vi "Dlg-Search-Stock.vi"(8 "error in (no error)":errorcluster) -> (0 "error out":errorcluster, 1 "Stock Selected":refnum<class "Stock.lvclass">, 2 "Canceled":bool, 3 "OK ?":bool)   [LabVIEW 2012]
uses:
  Stock Search.ctl
  Stock/Stock.lvclass
  Stock Manager Action.ctl
  Stock/Stock.lvclass/Stock.ctl
panel:
  in  "Stock":i32[](listbox)
  in  "Rechercher":string
  in  "Stock Search":T1
  in  "OK":bool
  out "Label":string
  in  "Cancel Button":bool
  # "Nouveau Portefeuille"
  # "Rechercher un Titre"
  # "Titre"
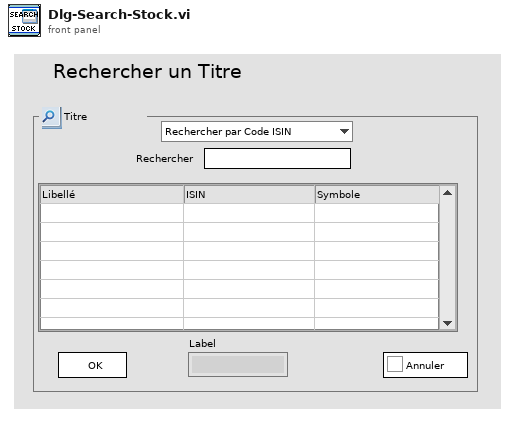
[diagram p1: front panel]
types:
  T1 = typedef "Stock Search.ctl" = enum16{"Rechercher par Code ISIN", "Rechercher par Libellé", "Rechercher par Symbole"}
  T2 = typedef "Stock Manager Action.ctl" = enum16{"Get_Stocks", "Load_Stocks", "Find_Stock_From_ISIN", "Find_Stock_From_Label", "Find_Stock_From_Symbol"}
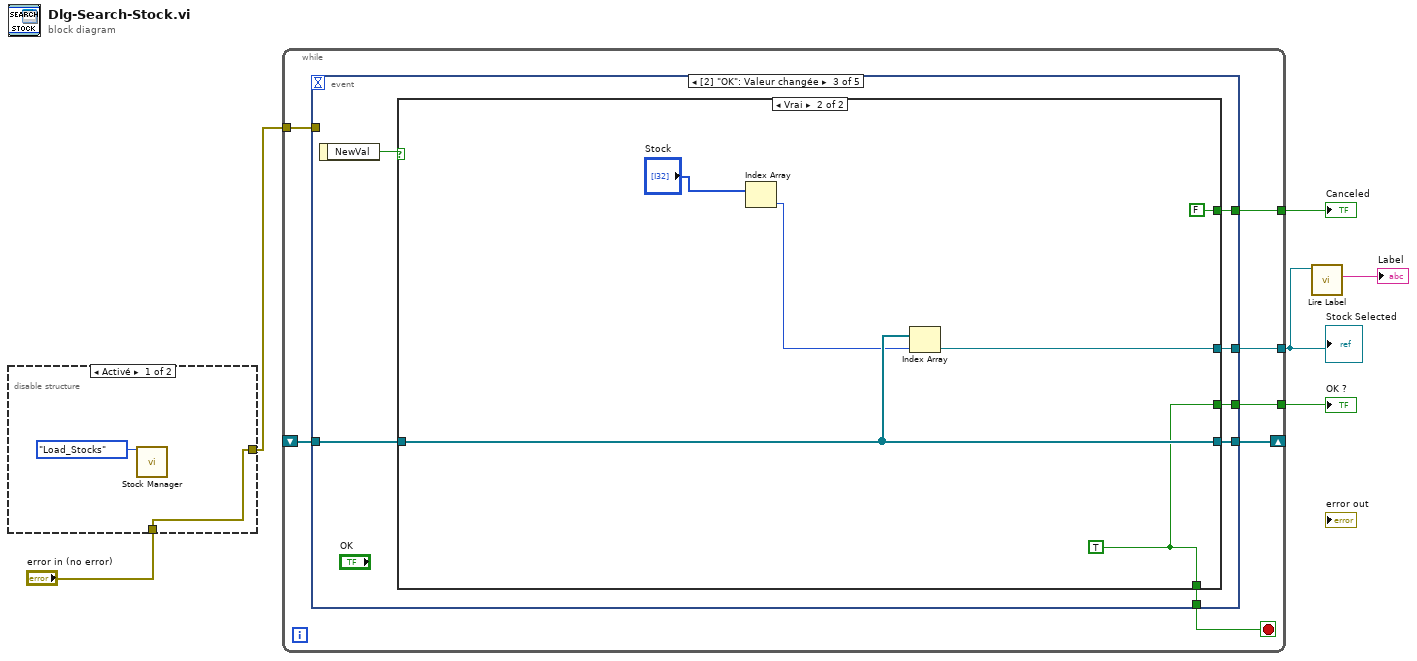
[diagram p0: block diagram]
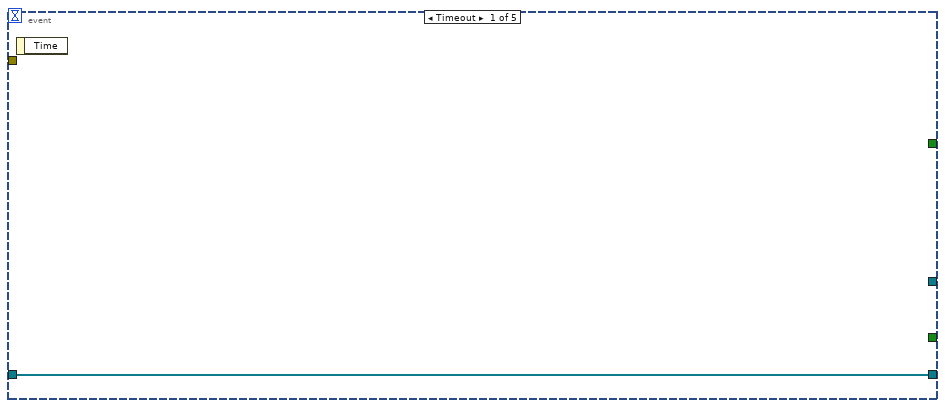
[diagram p2: hidden frame]
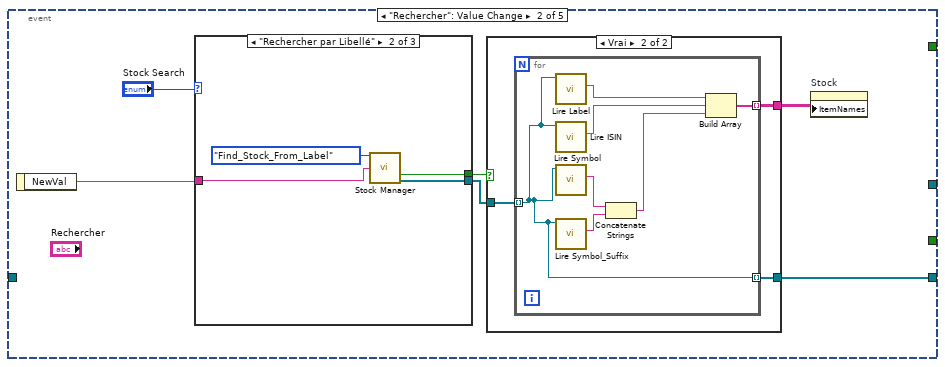
[diagram p3: hidden frame]
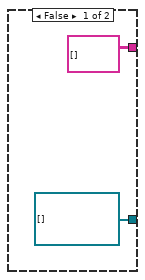
[diagram p4: hidden frame]
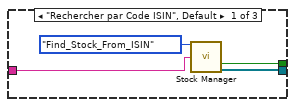
[diagram p5: hidden frame]
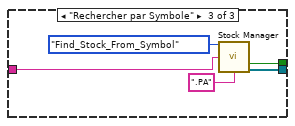
[diagram p6: hidden frame]
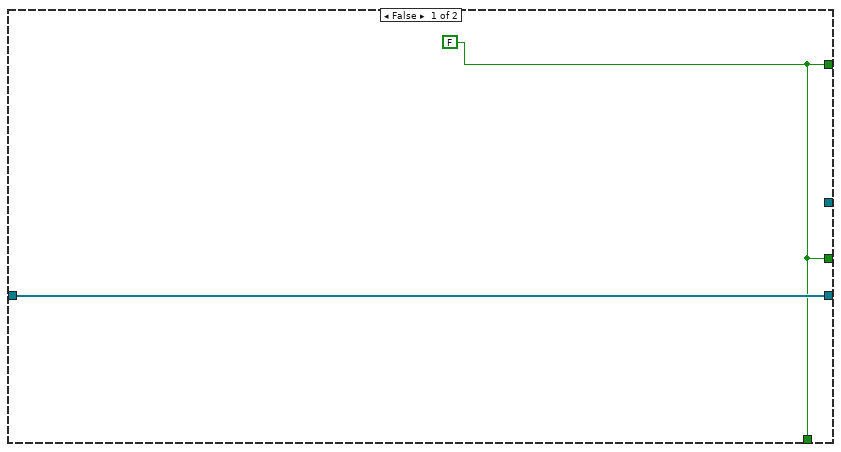
[diagram p7: hidden frame]
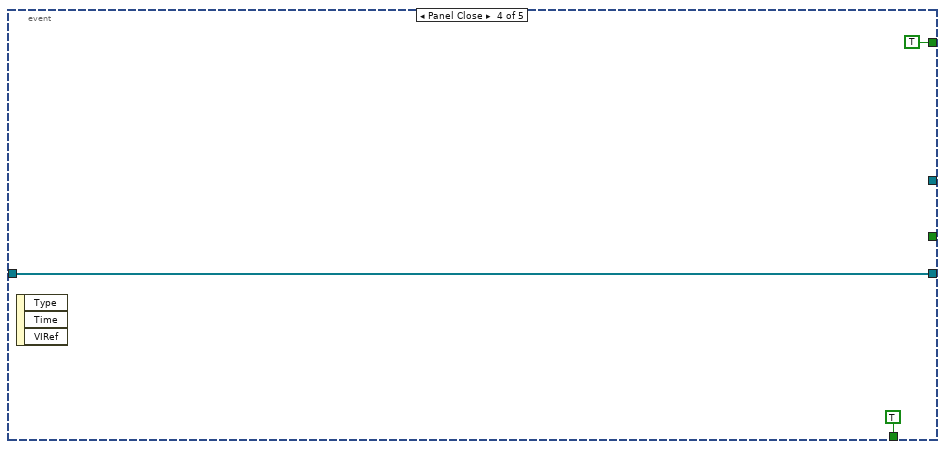
[diagram p8: hidden frame]
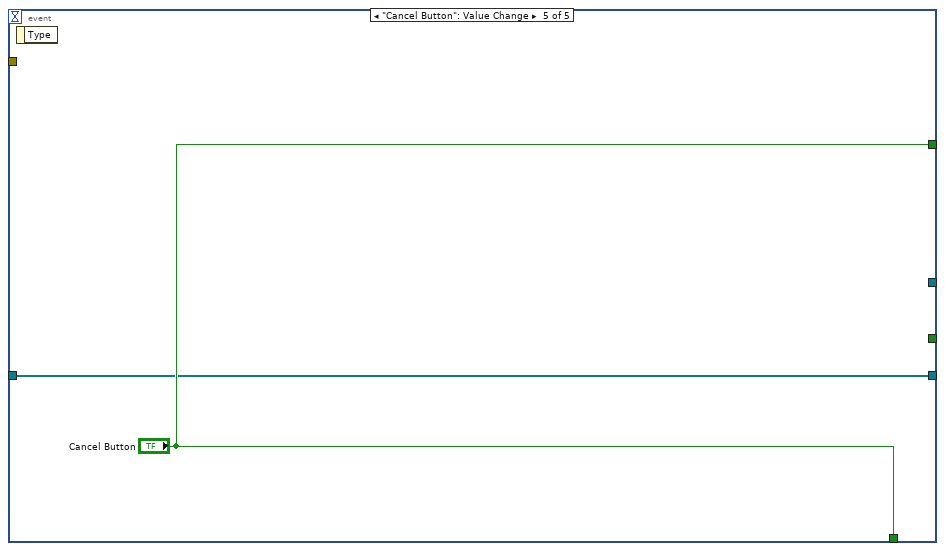
[diagram p9: hidden frame]
diagram:
  n1 = disable-structure shown="Activé" {
    disable-tunnel: [w7 _] -> w6
    disable-tunnel: "error in (no error)" -> [w7 _]
    frame Enabled {
      n2 = call "Stock Manager.vi"("Stock Manager Action"=Stock_Manager_Action."Load_Stocks") -> ()  [unwired: 12 in, 3 out]
    }
    frame Disabled {
    }
  }
  n3 = while {
    tunnel: w6 -> [w15]
    tunnel: [w14] -> w4
    shift-right: [w12] -> _
    shift-left: _ -> [w11]
    tunnel: [w10] -> w2
    tunnel: [w9] -> w3
    stop <- w13 stop-if-true
    n4 = event shown="[2] \"OK\": Valeur changée" {
      selector: _ -> [_ _ _ _ _]
      dyn-events: _ -> [_ _ _ _ _]
      timeout: _ -> [_ _ _ _ _]
      tunnel: w15 -> [_ _ _ _ _]
      tunnel: [_ _ w53 TRUE ("Cancel Button") "Cancel Button"] -> w14
      tunnel: [_ _ w52 TRUE ("Cancel Button") "Cancel Button"] -> w13
      tunnel: [w16 w17 w50 w63 w66] -> w12
      tunnel: w11 -> [w16 _ w51 w63 w66]
      tunnel: [_ _ w49 _ _] -> w10
      tunnel: [_ _ w48 _ _] -> w9
      event Timeout {
        n5 = event-data() -> ()  [unwired: 1 in, 1 out]
      }
      event "Rechercher": Value Change {
        n6 = event-data() -> ("NewVal"=w21:string)  [unwired: 1 in]
        n7 = case shown="\"Rechercher par Libellé\"" "Stock Search" {
          tunnel: w21 -> [w37 w41 w46]
          tunnel: [w36 w40 w44] -> w20
          tunnel: [w35 w39 w43] -> w19
          frame "Rechercher par Code ISIN", Default {
            n8 = call "Stock Manager.vi"("Stock Manager Action"=Stock_Manager_Action."Find_Stock_From_ISIN", "String to find (ISIN,Label,Symbol)"=w37) -> ("Stocks Found ?"=w36:bool, "Stocks Found"=w35:refnum<class "Stock.lvclass">[])  [unwired: 11 in, 1 out]
          }
          frame "Rechercher par Libellé" {
            n9 = call "Stock Manager.vi"("Stock Manager Action"=Stock_Manager_Action."Find_Stock_From_Label", "String to find (ISIN,Label,Symbol)"=w41) -> ("Stocks Found ?"=w40:bool, "Stocks Found"=w39:refnum<class "Stock.lvclass">[])  [unwired: 11 in, 1 out]
          }
          frame "Rechercher par Symbole" {
            n10 = call "Stock Manager.vi"("Stock Manager Action"=Stock_Manager_Action."Find_Stock_From_Symbol", "String to find (ISIN,Label,Symbol)"=w46, "Symbol_Suffix (.PA)"=".PA") -> ("Stocks Found ?"=w44:bool, "Stocks Found"=w43:refnum<class "Stock.lvclass">[])  [unwired: 10 in, 1 out]
          }
        }
        n11 = case shown="Vrai" w20 {
          tunnel: w19 -> [_ w27]
          tunnel: [string[][] [] w26] -> w18
          tunnel: [refnum<class "Stock.lvclass">[] [] w25] -> w17
          frame False {
          }
          frame True {
            n12 = for {
              tunnel: w27 -> [w28] mode=indexing
              tunnel: [w29] -> w26 mode=indexing
              tunnel: [w28] -> w25 mode=indexing
              n13 = call "Lire Label.vi"("Share en entrée"=w28) -> ("Label"=w32:string)  [unwired: 8 in, 2 out]
              n14 = call "Lire ISIN.vi"("Share en entrée"=w28) -> ("ISIN"=w31:string)  [unwired: 8 in, 2 out]
              n15 = call "Lire Symbol.vi"("Share en entrée"=w28) -> ("Symbol"=w34:string)  [unwired: 8 in, 2 out]
              n16 = call "Lire Symbol_Suffix.vi"("Stock en entrée"=w28) -> ("Symbol_Suffix"=w33:string)  [unwired: 8 in, 2 out]
              n17 = Concatenate Strings(w34, w33) -> (w30:string)
              n18 = Build Array(w32, w31, w30) -> (w29:string[])
            }
          }
        }
        n19 = property on="Stock" class="ListeMCol (strict)"("ItemNames"=w18) -> ()  [unwired: 2 in, 2 out]
      }
      event "OK": Value Change {
        n20 = event-data() -> ("NewVal"=w54:bool)  [unwired: 1 in]
        n21 = case shown="Vrai" w54 {
          tunnel: [w55 FALSE] -> w53
          tunnel: [w55 w57] -> w52
          tunnel: w51 -> [w56 w60]
          tunnel: [w56 w60] -> w50
          tunnel: [_ w58] -> w49
          tunnel: [w55 w57] -> w48
          frame False {
            w55 = FALSE
          }
          frame True {
            w57 = TRUE
            n22 = Index Array(array="Stock") -> (element=w59:i32)  [unwired: 1 in]
            n23 = Index Array(array=w60, index=w59) -> (element=w58:refnum<class "Stock.lvclass">)
          }
        }
      }
      event Panel Close {
        n24 = event-data() -> ()  [unwired: 1 in, 3 out]
      }
      event "Cancel Button": Value Change {
        n25 = event-data() -> ()  [unwired: 1 in, 1 out]
      }
    }
  }
  "Canceled" <- w4
  "Stock Selected" <- w2
  "OK ?" <- w3
  n26 = call "Lire Label.vi"("Share en entrée"=w2) -> ("Label"=→"Label":string)  [unwired: 8 in, 2 out]
